vi "SplitCode.vi"(10 "Code":string) -> (1 "BP Code":string, 2 "Spike Code":string)   [LabVIEW 2019]
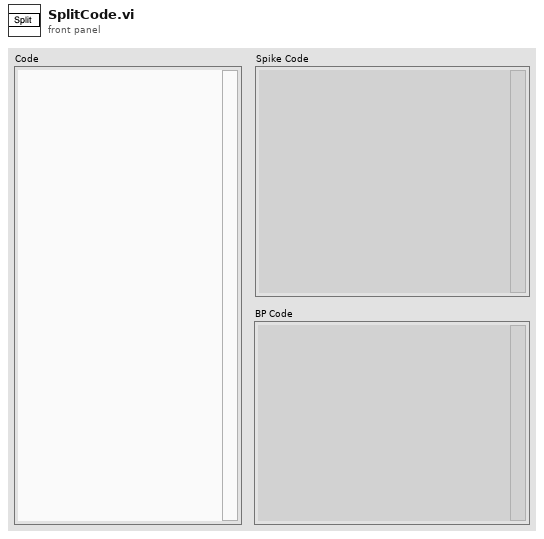
[diagram p1: front panel]
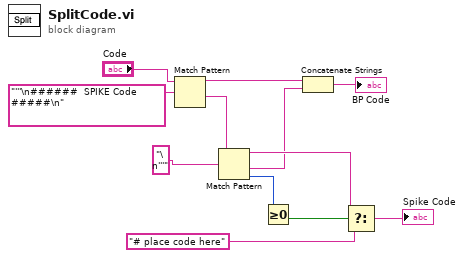
[diagram p0: block diagram]
diagram:
  n1 = Match Pattern(string="Code", regular expression="'''\n######  SPIKE Code #####\n") -> (before substring=w12:string, after substring=w8:string)  [unwired: 1 in, 2 out]
  n2 = Match Pattern(string=w8, regular expression="\n'''") -> (before substring=w9:string, after substring=w3:string, offset past match=w10:i32)  [unwired: 1 in, 1 out]
  n3 = Greater Or Equal To 0?(x=w10) -> (x >= 0?=w11:bool)
  n4 = Concatenate Strings(w12, w3) -> (→"BP Code":string)
  n5 = Select(t=w9, s=w11, f="# place code here") -> (s? t:f=→"Spike Code":string)
